vi "AIT 1553 - Separate Tx-Rx Messages.vi"(8 "error in (no error)":errorcluster, 11 "HW Channel - Section in":T1 {"Message Settings"."Driver Data"."First Word" min=8 max=31; "Message Settings"."Driver Data"."Num Bits" min=1 max=32; "Message Settings"."Driver Data"."Start Bit" min=8 max=31; "Message Settings"."Block Data Refs"."Data Reference" format="%.0x"}) -> (0 "error out":errorcluster, 2 "HW Channel Rx - Section out":T1 {"Message Settings"."Driver Data"."First Word" min=8 max=31; "Message Settings"."Driver Data"."Num Bits" min=1 max=32; "Message Settings"."Driver Data"."Start Bit" min=8 max=31; "Message Settings"."Block Data Refs"."Data Reference" format="%.0x"}, 3 "HW Channel Tx - Section out":T1 {"Message Settings"."Driver Data"."First Word" min=8 max=31; "Message Settings"."Driver Data"."Num Bits" min=1 max=32; "Message Settings"."Driver Data"."Start Bit" min=8 max=31; "Message Settings"."Block Data Refs"."Data Reference" format="%.0x"})   [LabVIEW 2014, in "AIT 1553 Custom Device.lvlib"]
uses:
  AIT 1553 Custom Device.lvlib
  RT Controls/AIT 1553 - RT HW Channel.ctl
  RT Controls/AIT 1553 - Bus Section.ctl
  RT Controls/AIT 1553 - RT Message Settings.ctl
  <vilib>/NI Veristand/Custom Device API/Block Data Reference.ctl
  <vilib>/NI Veristand/Custom Device API/Data Reference.ctl
  RT Controls/AIT 1553 - Driver Data.ctl
  Controls and Global/Start Bit.ctl
  Controls and Global/Number of Bits.ctl
  <vilib>/NI Veristand/Custom Device API/Custom Device API.lvlib
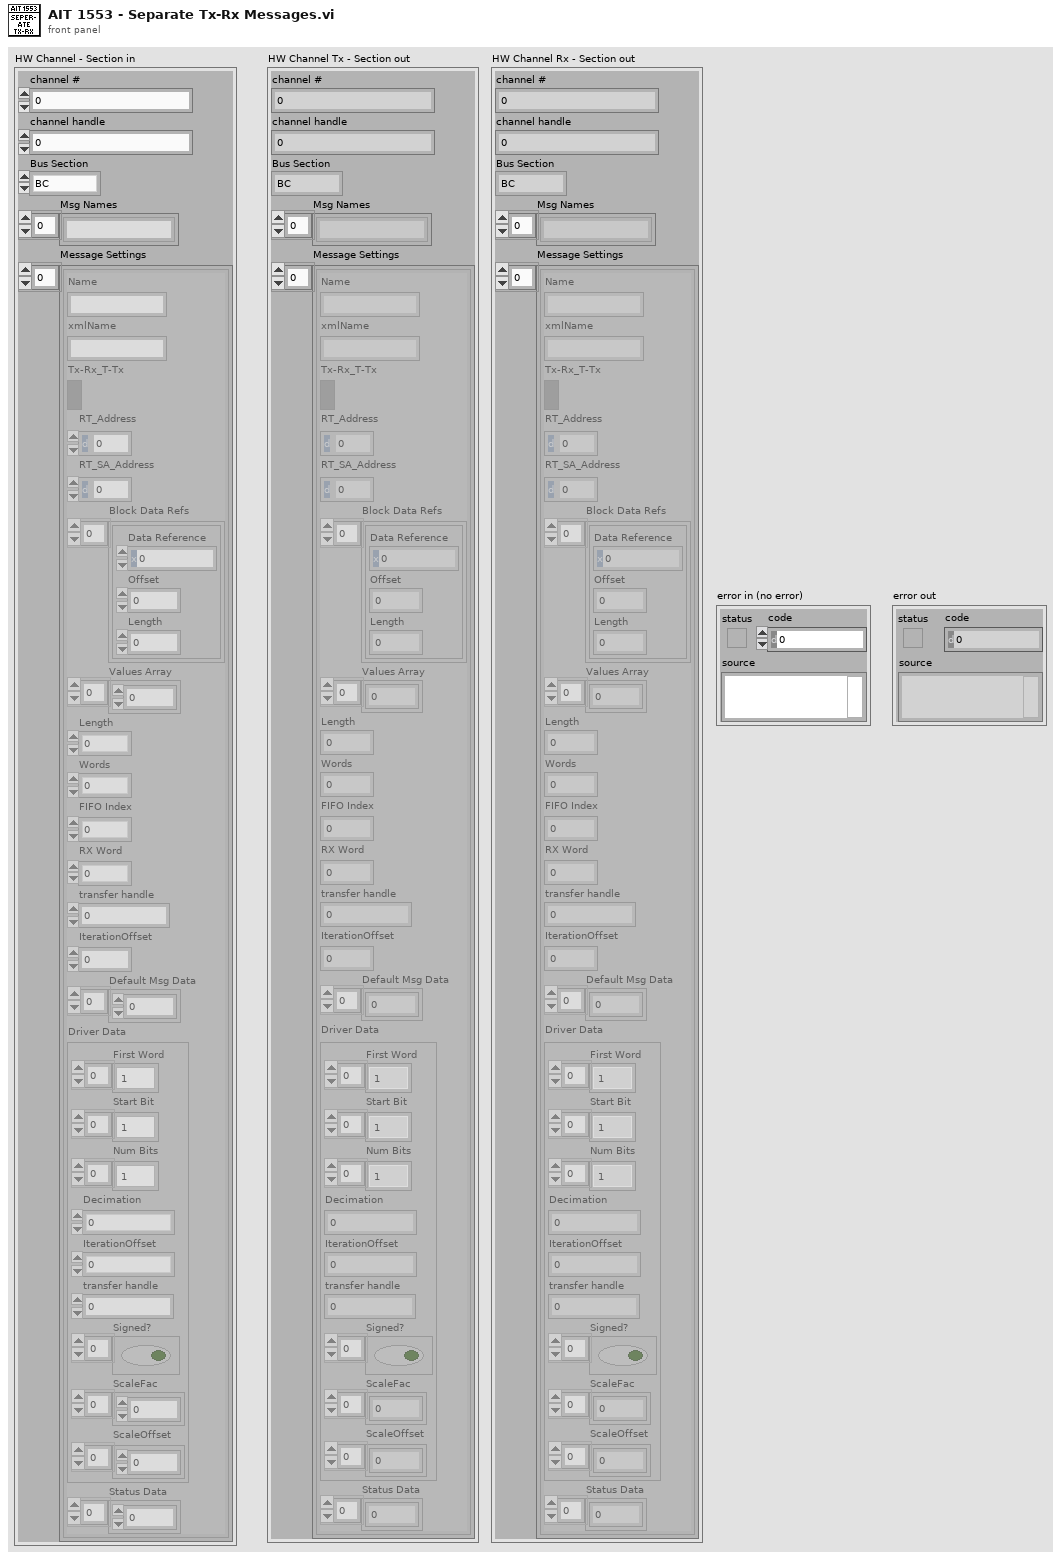
[diagram p1: front panel]
types:
  T1 = typedef "AIT 1553 Custom Device.lvlib/AIT 1553 - RT HW Channel.ctl" = cluster{"channel #":u16, "channel handle":u32, "Bus Section":T2, "Msg Names":string[], "Message Settings":T3[]}
  T2 = typedef "AIT 1553 Custom Device.lvlib/AIT 1553 - Bus Section.ctl" = enum16{"BC", "BM", "RT"}
  T3 = typedef "AIT 1553 Custom Device.lvlib/AIT 1553 - RT Message Settings.ctl" = cluster{"Name":string, "xmlName":string, "Tx-Rx_T-Tx":bool, "RT_Address":u8, "RT_SA_Address":u8, "Block Data Refs":T4[], "Values Array":dbl[], "Length":i32, "Words":i32, "FIFO Index":i32, "RX Word":u32, "transfer handle":u32, "IterationOffset":i32, "Default Msg Data":u16[], "Driver Data":T6, "Status Data":u32[]}
  T4 = typedef "Custom Device API.lvlib/Block Data Reference.ctl" = cluster{"Data Reference":T5, "Offset":i32, "Length":i32}
  T5 = typedef "Custom Device API.lvlib/Data Reference.ctl" = i32
  T6 = typedef "AIT 1553 Custom Device.lvlib/AIT 1553 - Driver Data.ctl" = cluster{"First Word":T7[], "Start Bit":T7[], "Num Bits":T8[], "Decimation":i32, "IterationOffset":i32, "transfer handle":u32, "Signed?":bool[], "ScaleFac":dbl[], "ScaleOffset":dbl[]}
  T7 = typedef "AIT 1553 Custom Device.lvlib/Start Bit.ctl" = i32
  T8 = typedef "AIT 1553 Custom Device.lvlib/Number of Bits.ctl" = i32
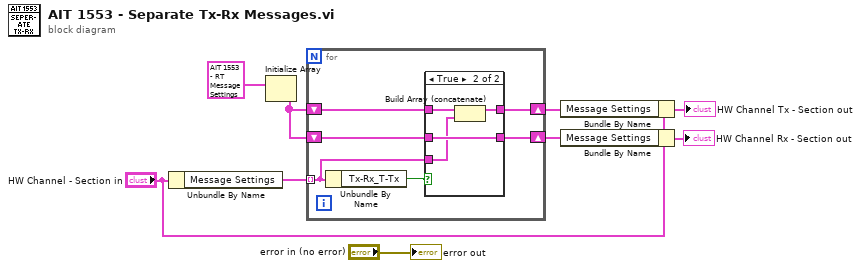
[diagram p0: block diagram]
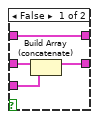
[diagram p2: hidden frame]
diagram:
  n1 = Unbundle By Name("HW Channel - Section in") -> ("Message Settings"=w3:T3[])
  n2 = Initialize Array(T3 {"Name"="", "xmlName"="", "Tx-Rx_T-Tx"=FALSE, "RT_Address"=0, "RT_SA_Address"=0, "Block Data Refs"=[], "Values Array"=[], "Length"=0, "Words"=0, "FIFO Index"=0, "RX Word"=0, "transfer handle"=0, "IterationOffset"=0, "Default Msg Data"=[], "Driver Data"={"First Word"=[], "Start Bit"=[], "Num Bits"=[], "Decimation"=0, "IterationOffset"=0, "transfer handle"=0, "Signed?"=[], "ScaleFac"=[], "ScaleOffset"=[]}, "Status Data"=[]} ("Message Settings")) -> (w5:T3[])  [unwired: 1 in]
  n3 = for {
    shift-right: [w10] -> w8
    shift-left: w5 -> [w13]
    shift-right: [w11] -> w7
    shift-left: w5 -> [w12]
    tunnel: w3 -> [w14] mode=indexing
    n4 = Unbundle By Name(w14) -> ("Tx-Rx_T-Tx"=w15:bool)
    n5 = case shown="True" w15 {
      tunnel: w14 -> [w18 w21]
      tunnel: w13 -> [w17 w22]
      tunnel: w12 -> [w19 w23]
      tunnel: [w16 w23] -> w11
      tunnel: [w17 w20] -> w10
      frame False {
        n6 = Build Array (concatenate)(w19, w18) -> (w16:T3[])
      }
      frame True {
        n7 = Build Array (concatenate)(w22, w21) -> (w20:T3[])
      }
    }
  }
  n8 = Bundle By Name(cluster="HW Channel - Section in", "Message Settings"=w8) -> (→"HW Channel Tx - Section out":T1)
  n9 = Bundle By Name(cluster="HW Channel - Section in", "Message Settings"=w7) -> (→"HW Channel Rx - Section out":T1)
  "error out" <- "error in (no error)"
